vi "execute.vi"(8 "error in (no error)":errorcluster, 10 "Context in":refnum<class "Context.lvclass">, 11 "MoveHardpointActuatorsCommand in":refnum<class "MoveHardpointActuatorsCommand.lvclass">) -> (0 "error out":errorcluster, 2 "Context out":refnum<class "Context.lvclass">, 3 "MoveHardpointActuatorsCommand out":refnum<class "MoveHardpointActuatorsCommand.lvclass">)   [LabVIEW 2016, in "MoveHardpointActuatorsCommand.lvclass"]
uses:
  MoveHardpointActuatorsCommand.lvclass
  Context/Context.lvclass
  MoveHardpointActuatorsCommand.lvclass/MoveHardpointActuatorsCommand.ctl
  Context/Context.lvclass/Context.ctl
  Context/getModel.vi
  Context/setModel.vi
  Model/getState.vi
  States/State/State.lvclass
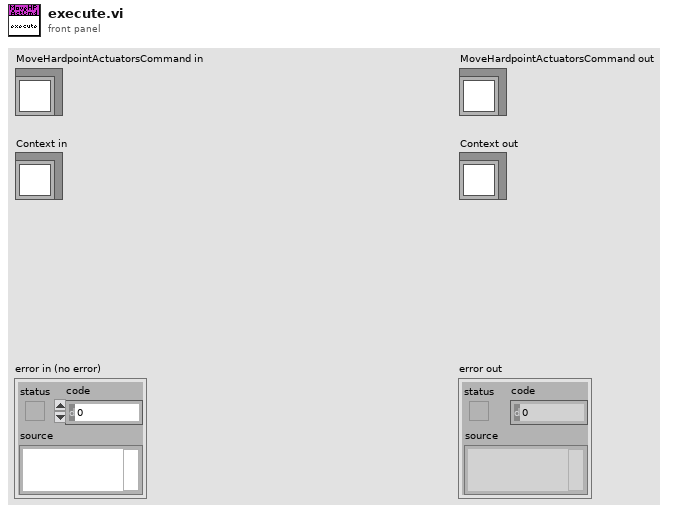
[diagram p1: front panel]
types:
  T1 = typedef "M1M3SupportTopics.lvlib/CommandMoveHardpointActuators.ctl" = cluster{"CommandId":T2, "Steps":i8[]}
  T2 = typedef "M1M3SupportTopics.lvlib/CommandId.ctl" = i32
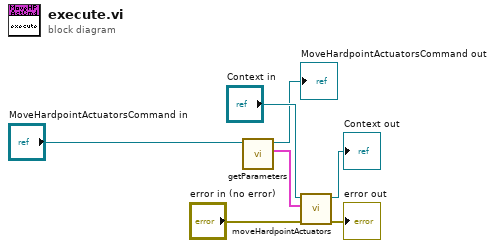
[diagram p0: block diagram]
diagram:
  n1 = call "getParameters.vi"("MoveHardpointActuatorsCommand in"="MoveHardpointActuatorsCommand in") -> ("Parameters"=w1:T1, "MoveHardpointActuatorsCommand out"=→"MoveHardpointActuatorsCommand out":refnum<class "MoveHardpointActuatorsCommand.lvclass">)  [unwired: 9 in]
  n2 = call "moveHardpointActuators.vi"("error in (no error)"="error in (no error)", "Parameters"=w1, "Context in"="Context in") -> ("error out"=→"error out":errorcluster, "Context out"=→"Context out":refnum<class "Context.lvclass">)  [unwired: 7 in]
